vi "Needs Expension.vi"(7 "Grid Size":i32[](array[numeric]), 11 "Points In":set{cluster{i32, i32}}(c389)) -> (3 "Expension Directions":enum16{"Left", "Right", "Up", "Down"}[](array[ring]))   [LabVIEW 2021]
uses:
  f498c2b4-f735-4c7d-b7b5-6f4f1d763306.vi
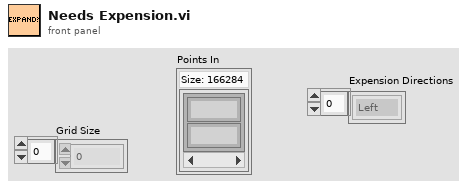
[diagram p1: front panel]
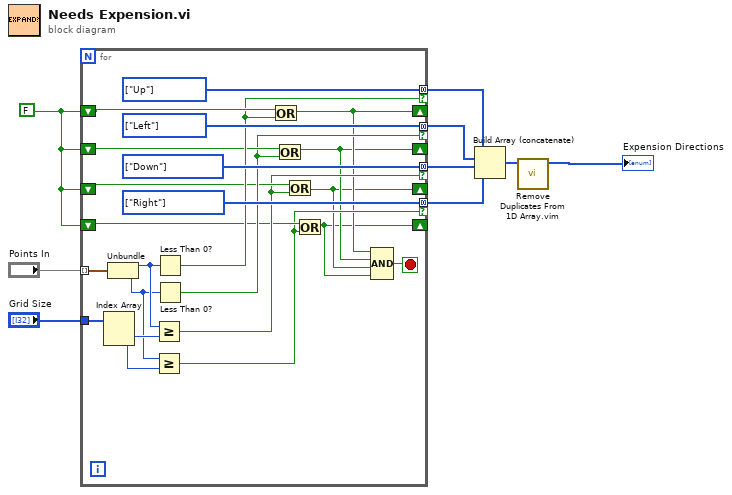
[diagram p0: block diagram]
diagram:
  w1 = FALSE
  n1 = for {
    tunnel: "Points In" -> [w32] mode=indexing
    tunnel: "Grid Size" -> [w30]
    tunnel: [w26] -> w6 mode=concatenating if=w21
    tunnel: [w25] -> w4 mode=concatenating if=w19
    tunnel: [w24] -> w5 mode=concatenating if=w17
    tunnel: [w23] -> w7 mode=concatenating if=w15
    shift-right: [w14] -> _
    shift-left: w1 -> [w22]
    shift-right: [w13] -> _
    shift-left: w1 -> [w20]
    shift-right: [w12] -> _
    shift-left: w1 -> [w18]
    shift-right: [w11] -> _
    shift-left: w1 -> [w16]
    stop <- w10 stop-if-true
    w23 = enum16{"Left", "Right", "Up", "Down"}[] [enum."Right"] items=["Left", "Right", "Up", "Down"] ("Expension Directions")
    w24 = enum16{"Left", "Right", "Up", "Down"}[] [enum."Down"] items=["Left", "Right", "Up", "Down"] ("Expension Directions")
    w25 = enum16{"Left", "Right", "Up", "Down"}[] [enum."Left"] items=["Left", "Right", "Up", "Down"] ("Expension Directions")
    w26 = enum16{"Left", "Right", "Up", "Down"}[] [enum."Up"] items=["Left", "Right", "Up", "Down"] ("Expension Directions")
    n2 = Index Array(array=w30) -> (element #1=w29:i32, element #2=w27:i32)  [unwired: 2 in]
    n3 = Unbundle(w32) -> (w31:i32, w28:i32)
    n4 = Greater Or Equal?(x=w31, y=w29) -> (x >= y?=w17:bool)
    n5 = Greater Or Equal?(x=w28, y=w27) -> (x >= y?=w15:bool)
    n6 = Less Than 0?(x=w31) -> (x < 0?=w21:bool)
    n7 = Less Than 0?(x=w28) -> (x < 0?=w19:bool)
    n8 = Or(x=w22, y=w21) -> (x .or. y?=w14:bool)
    n9 = Or(x=w20, y=w19) -> (x .or. y?=w13:bool)
    n10 = Or(x=w18, y=w17) -> (x .or. y?=w12:bool)
    n11 = Or(x=w16, y=w15) -> (x .or. y?=w11:bool)
    n12 = Compound Arithmetic op=AND(w14, w13, w12, w11) -> (w10:bool)
  }
  n13 = Build Array (concatenate)(w6, w4, w5, w7) -> (w3:enum16{"Left", "Right", "Up", "Down"}[])
  n14 = call "Remove Duplicates From 1D Array.vim"("array"=w3) -> ("array with duplicates removed"=→"Expension Directions":enum16{"Left", "Right", "Up", "Down"}[])  [unwired: 10 in]
